vi "DriveControlManager.vi"(0 "Left Drive Manual Control":dbl, 1 "Right Drive Manual Control":dbl, 2 "left drive unit conversion (ticks/in)":dbl, 3 "right drive unit coversion (ticks/in)":dbl, 4 "LeftTrajectory":T1[](array[typedef]), 5 "RightTrajectory":T1[](array[typedef]), 6 "StartAtZero":bool=TRUE, 8 "Right Drive Motor DevRef":T3={"DeviceStatus"={"status"=FALSE, "code"=0, "source"=""}, "Type"=enum."PWM", "PWM"={"PWM Channel"=enum."PWM 1", "DeadBand"={"Name"="", "maxPositivePwm"=0, "minPositivePwm"=0, "centerPwm"=0, "maxNegativePwm"=0, "minNegativePwm"=0, "angularRange"=0}}, "CAN"={"Device Number"=0, "SetOutput VI Ref"=variant(enum8{"Percent VBus", "Current", "Speed", "Position", "Voltage"} enum."Percent VBus"), "GetOutput VI Ref"=variant(refnum<k1> refnum), "Enable VI Ref"=variant(dbl 12.0), "Disable VI Ref"=variant(enum8{"Percent VBus", "Speed", "Position", "Slave", "Unchanged / Invalid", "Voltage Compensation", "Current", "Motion Profile"} enum."Percent VBus"), "Data"=variant}, "Invert"=FALSE, "DIO PWM"={"PWM \"Enable\" Channel"=enum."Invalid", "DIOChannel"=enum."Invalid", "PWM Rate"=0.0}}, 9 "New Motion Profile":bool, 10 "Left Drive Motor DevRef":T3={"DeviceStatus"={"status"=FALSE, "code"=0, "source"=""}, "Type"=enum."PWM", "PWM"={"PWM Channel"=enum."PWM 1", "DeadBand"={"Name"="", "maxPositivePwm"=0, "minPositivePwm"=0, "centerPwm"=0, "maxNegativePwm"=0, "minNegativePwm"=0, "angularRange"=0}}, "CAN"={"Device Number"=0, "SetOutput VI Ref"=variant(enum8{"Percent VBus", "Current", "Speed", "Position", "Voltage"} enum."Percent VBus"), "GetOutput VI Ref"=variant(refnum<k1> refnum), "Enable VI Ref"=variant(dbl 12.0), "Disable VI Ref"=variant(enum8{"Percent VBus", "Speed", "Position", "Slave", "Unchanged / Invalid", "Voltage Compensation", "Current", "Motion Profile"} enum."Percent VBus"), "Data"=variant}, "Invert"=FALSE, "DIO PWM"={"PWM \"Enable\" Channel"=enum."Invalid", "DIOChannel"=enum."Invalid", "PWM Rate"=0.0}}) -> (14 "Drive Control State":T2)   [LabVIEW 2017]
uses:
  General/MotionProfiling/TypeDefs/MotionProfileControlState.ctl
  <vilib>/Rock Robotics/WPI/MotorControl/WPI_MotorControlDeviceRef.ctl
  <vilib>/Rock Robotics/WPI/MotorControl/WPI_MotorControlType.ctl
  <vilib>/Rock Robotics/SystemInterfaces/DIO/FPGA_DIOPWMChannel.ctl
  <vilib>/Rock Robotics/WPI/PWM/WPI_PWMDeadband.ctl
  <vilib>/Rock Robotics/SystemInterfaces/DIO/FPGA_DIOChannel.ctl
  Pathfinder/Pathfinder-LabVIEW/Pathfinder-Lib/VIs/Segment.ctl
  <vilib>/Rock Robotics/WPI/DriverStation/WPI_DriverStationRobotMode2.ctl
  ArgosLib/Signal Processing/TypeDefs/EdgeDetector_Type.ctl
  <vilib>/Rock Robotics/WPI/ThirdParty/Phoenix-LabVIEW/Motor Controller/Controls/CTRE_Phoenix_MotorControl_ControlMode.ctl
  Global_Var-RefNum/MotionProfileControlData.vi
  <vilib>/Rock Robotics/WPI/ThirdParty/Phoenix-LabVIEW/Motor Controller/Get/CTRE_Phoenix_MotorController_GetSelectedSensorData.vi
  <vilib>/Rock Robotics/WPI/ThirdParty/Phoenix-LabVIEW/Motor Controller/Get/CTRE_Phoenix_MotorController_GetClosedLoopData.vi
  <vilib>/Rock Robotics/WPI/ThirdParty/Phoenix-LabVIEW/Motor Controller/Get/CTRE_Phoenix_MotorController_GetVoltage.vi
  ArgosLib/ArgosLib.lvlib
  Pathfinder/Pathfinder-LabVIEW/Pathfinder-Lib/Pathfinder.lvlib
panel:
  in  "StopDetectTime (ms)":u32
  in  "Tab Control":enum32{"I/O", "Calibration", "Status"}(tab)
  in  "ClearMotionProfile":bool
  out "Max Left Drive Speed (Sensor Units per 100 ms)":i32
  out "Max Right Drive Speed (Sensor Units per 100 ms)":i32
  in  "Reset Right Drive Max":bool
  in  "Reset Left Drive Max":bool
  in  "Reset Left Drive Sensor":bool
  in  "Reset Right Drive Sensor":bool
  in  "Left Drive Position (in)":dbl
  in  "Right Drive Position (in)":dbl
  out "Left Drive":T8
  out "Right Drive":T8
  out "RightDriveFaults":T9
  out "LeftDriveFaults":T9
  out "Right Error":i32
  out "Left Error":i32
  out "LeftDriveV":dbl(graph)
  out "RightDriveV":dbl(graph)
  out "Right Drive":T8(graph)
  out "Left Drive":T8(graph)
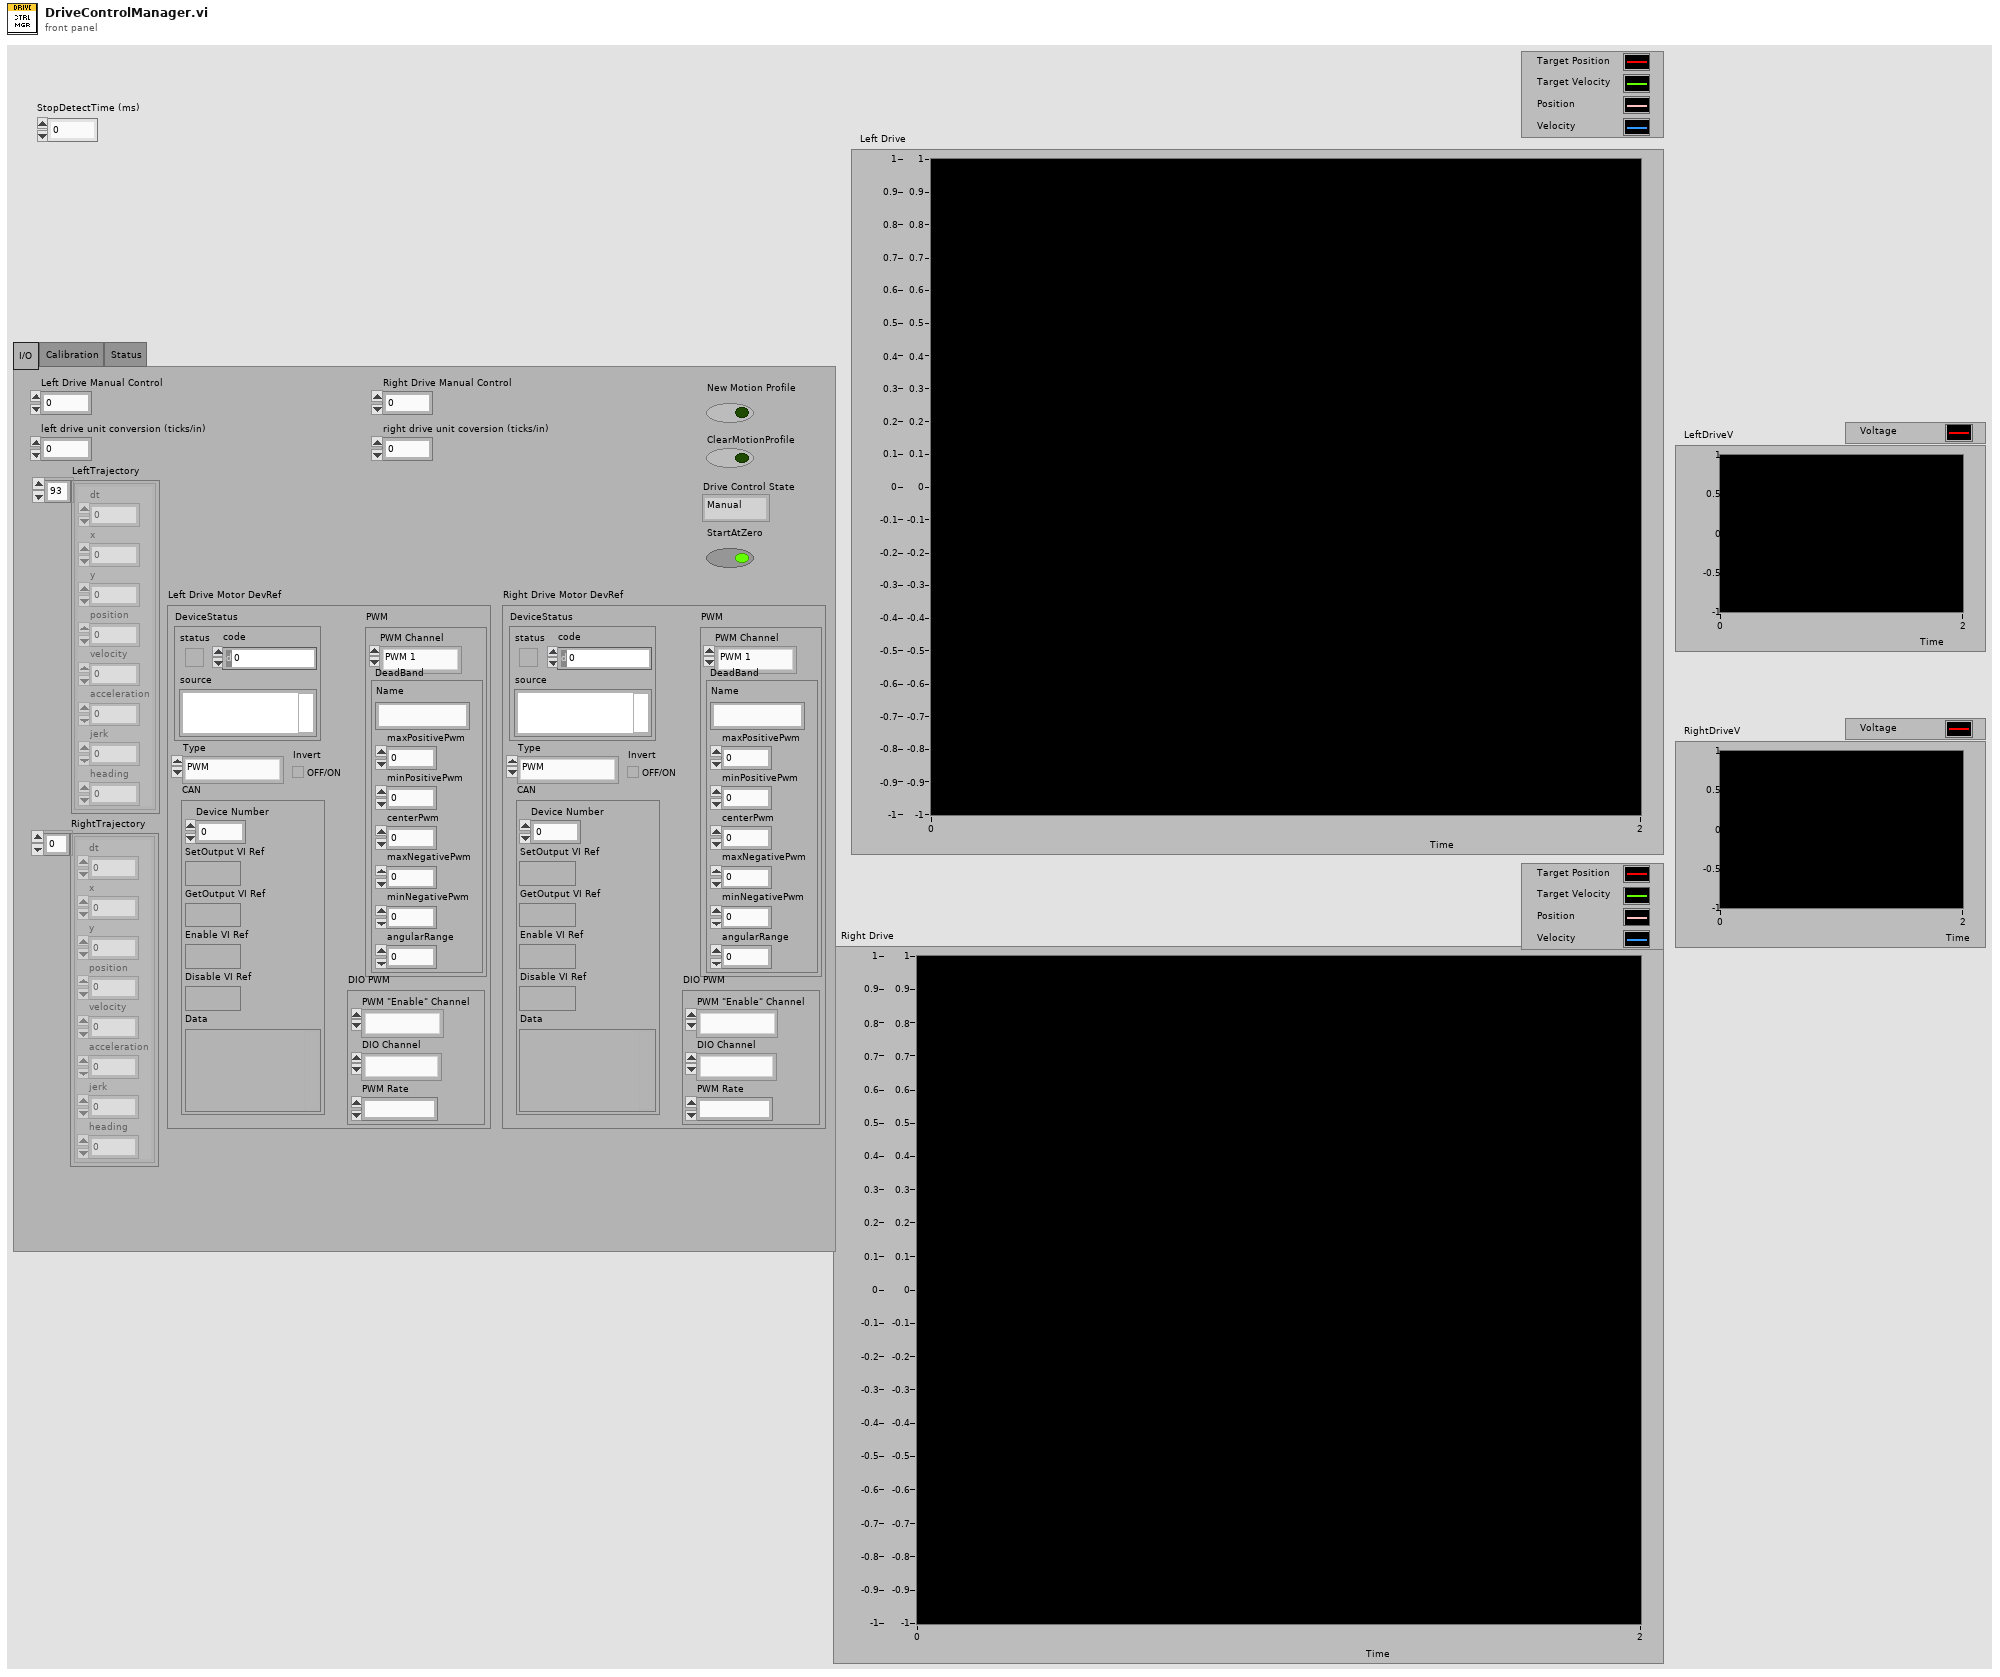
[diagram p1: front panel]
types:
  T1 = typedef "Pathfinder.lvlib/Segment.ctl" = cluster{"dt":dbl, "x":dbl, "y":dbl, "position":dbl, "velocity":dbl, "acceleration":dbl, "jerk":dbl, "heading":dbl}
  T2 = typedef "MotionProfileControlState.ctl" = enum16{"Manual", "Auto_Idle", "Auto_Run"}
  T3 = typedef "WPI_MotorControlDeviceRef.ctl" = cluster{"DeviceStatus":errorcluster, "Type":T4, "PWM":cluster{"PWM Channel":T5, "DeadBand":T6}, "CAN":cluster{"Device Number":u8, "SetOutput VI Ref":variant, "GetOutput VI Ref":variant, "Enable VI Ref":variant, "Disable VI Ref":variant, "Data":variant}, "Invert":bool, "DIO PWM":cluster{"PWM \"Enable\" Channel":T5, "DIOChannel":T7, "PWM Rate":dbl}}
  T4 = typedef "WPI_MotorControlType.ctl" = enum16{"PWM", "CAN", "DIO PWM"}
  T5 = typedef "FPGA_DIOPWMChannel.ctl" = enum8{"PWM 0", "PWM 1", "PWM 2", "PWM 3", "PWM 4", "PWM 5", "PWM 6", "PWM 7", "PWM 8", "PWM 9", "PWM MXP 0", "PWM MXP 1", "PWM MXP 2", "PWM MXP 3", "PWM MXP 4", "PWM MXP 5", "PWM MXP 6", "PWM MXP 7", "PWM MXP 8", "PWM MXP 9", "Invalid"}
  T6 = typedef "WPI_PWMDeadband.ctl" = cluster{"Name":string, "maxPositivePwm":i32, "minPositivePwm":i32, "centerPwm":i32, "maxNegativePwm":i32, "minNegativePwm":i32, "angularRange":u16}
  T7 = typedef "FPGA_DIOChannel.ctl" = enum8{"DIO 0", "DIO 1", "DIO 2", "DIO 3", "DIO 4", "DIO 5", "DIO 6", "DIO 7", "DIO 8", "DIO 9", "DIO MXP 0", "DIO MXP 1", "DIO MXP 2", "DIO MXP 3", "DIO MXP 4", "DIO MXP 5", "DIO MXP 6", "DIO MXP 7", "DIO MXP 8", "DIO MXP 9", "DIO MXP 10", "DIO MXP 11", "DIO MXP 12", "DIO MXP 13", "DIO MXP 14", "DIO MXP 15", "SPI Port CS1", "SPI Port CS2", "SPI Port CS3", "SPI Port MISO", "SPI Port MOSI", "Invalid"}
  T8 = cluster{"Position (Sensor Units)":i32, "Velocity (Sensor Units per 100 ms)":i32, "Position (Raw Sensor Units)":i32, "Velocity (Raw Sensor Units per 100 ms)":i32}
  T9 = cluster{"Under Voltage":bool, "Forward Limit Switch":bool, "Reverse Limit Switch":bool, "Forward Soft Limit":bool, "Reverse Soft Limit":bool, "Hardware Failure":bool, "Reset During Enable":bool, "Sensor Overflow":bool, "Sensor Out of Phase":bool, "Hardware ESD Reset":bool, "Remote Loss of Signal":bool}
  T10 = typedef "WPI_DriverStationRobotMode2.ctl" = enum16{"Autonomous Disabled", "Autonomous Enabled", "Teleop Disabled", "Teleop Enabled", "Disconnected", "Finish", "Test Disabled", "Test Enabled", "Emergency Stopped"}
  T11 = typedef "ArgosLib.lvlib/EdgeDetector_Type.ctl" = enum16{"RisingEdge", "FallingEdge", "Both"}
  T12 = cluster{"Position (Sensor Units)":i32, "Velocity (Sensor Units per 100 ms)":i32, "Position (Raw Sensor Units)":i32, "Velocity (Raw Sensor Units per 100 ms)":i32}[]
  T13 = typedef "CTRE_Phoenix_MotorControl_ControlMode.ctl" = u16
  T14 = typedef "DriveMotionProfileControl.ctl" = cluster{"ControlMutex":T15, "Trajectory Points":T1[], "CurrentIndex":u32}
  T15 = typedef "Semaphore RefNum" = refnum<k1>
  T16 = cluster{"Position (Raw Sensor Units)":i32, "Closed-loop Target":i32, "Position (Raw Sensor Units)":i32, "Velocity (Raw Sensor Units per 100 ms)":i32}
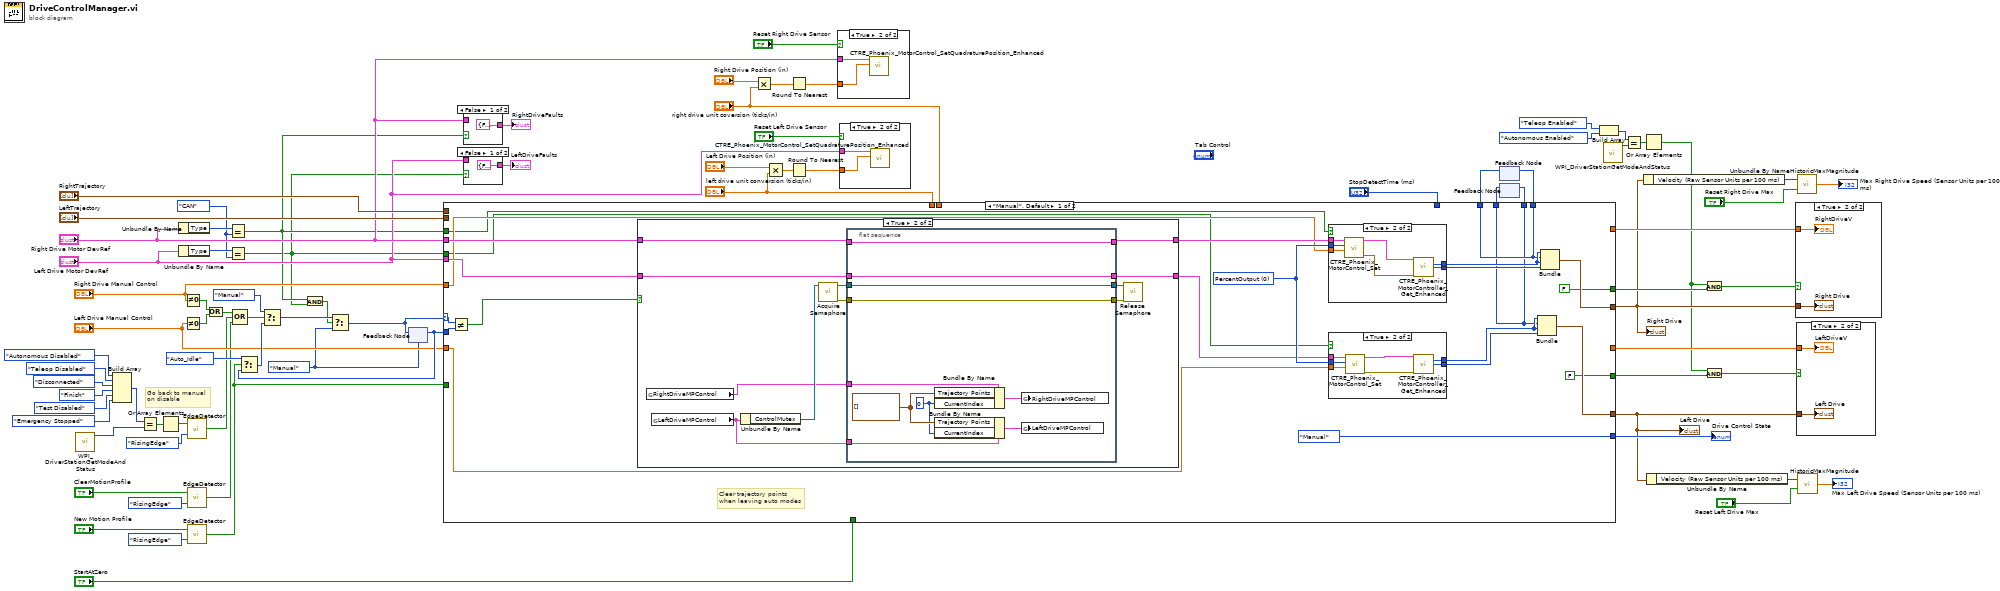
[diagram p0: block diagram]
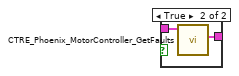
[diagram p2: hidden frame]
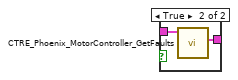
[diagram p3: hidden frame]
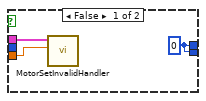
[diagram p8: hidden frame]
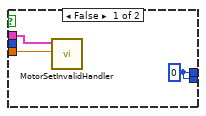
[diagram p9: hidden frame]
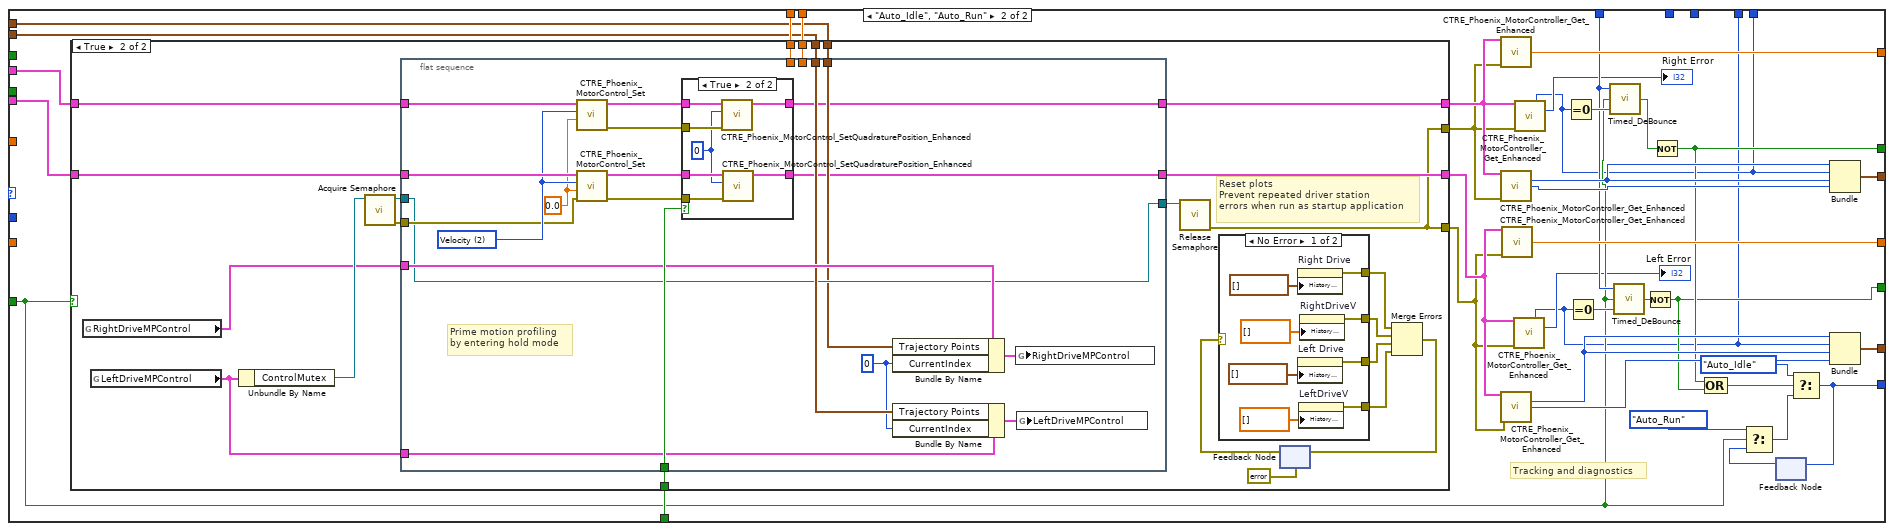
[diagram p11: hidden frame]
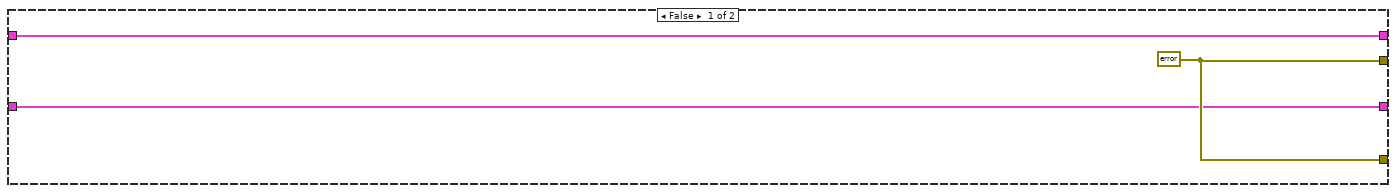
[diagram p12: hidden frame]
diagram:
  w4 = MotionProfileControlState."Manual" ("f")
  w7 = WPI_MotorControlType."CAN" ("y")
  # "Go back to manual\non disable"
  n1 = call <vilib>:"WPI_DriverStationGetModeAndStatus.vi"() -> ("Robot Mode"=w39:T10)  [unwired: 10 in, 1 out]
  n2 = Build Array(WPI_DriverStationRobotMode2."Autonomous Disabled" ("Robot Mode"), WPI_DriverStationRobotMode2."Teleop Disabled" ("Robot Mode"), WPI_DriverStationRobotMode2."Disconnected" ("Robot Mode"), WPI_DriverStationRobotMode2."Finish" ("Robot Mode"), WPI_DriverStationRobotMode2."Test Disabled" ("Robot Mode"), WPI_DriverStationRobotMode2."Emergency Stopped" ("Robot Mode")) -> (w40:T10[])
  n3 = Equal?(x=w40, y=w39) -> (x = y?=w38:bool[])
  n4 = Or Array Elements(Boolean array=w38) -> (logical OR=w37:bool)
  n5 = Unbundle By Name("Right Drive Motor DevRef") -> ("Type"=w9:T4)
  n6 = Unbundle By Name("Left Drive Motor DevRef") -> ("Type"=w8:T4)
  n7 = Not Equal To 0?(x="Right Drive Manual Control") -> (x != 0?=w80:bool)
  n8 = Not Equal To 0?(x="Left Drive Manual Control") -> (x != 0?=w79:bool)
  n9 = call "EdgeDetector.vi"("DetectorType"=EdgeDetector_Type."RisingEdge", "Input"=w37) -> ("Edge"=w34:bool)
  n10 = call "EdgeDetector.vi"("DetectorType"=EdgeDetector_Type."RisingEdge", "Input"="ClearMotionProfile") -> ("Edge"=w35:bool)
  n11 = call "EdgeDetector.vi"("DetectorType"=EdgeDetector_Type."RisingEdge", "Input"="New Motion Profile") -> ("Edge"=w72:bool)
  n12 = Or(x=w80, y=w79) -> (x .or. y?=w55:bool)
  n13 = Equal?(x=w9, y=w7) -> (x = y?=w2:bool)
  n14 = Equal?(x=w8, y=w7) -> (x = y?=w1:bool)
  n15 = Compound Arithmetic op=OR(w55, w34, w35) -> (w56:bool)
  n16 = And(x=w2, y=w1) -> (x .and. y?=w3:bool)
  n17 = feedback #1(w4) -> (w76:T2)
  n18 = Select(t=MotionProfileControlState."Auto_Idle", s=w72, f=w76) -> (s? t:f=w77:T2)
  n19 = Select(t=MotionProfileControlState."Manual" ("Arm Control State"), s=w56, f=w77) -> (s? t:f=w6:T2)
  n20 = Select(t=w6, s=w3, f=w4) -> (s? t:f=w5:T2)
  n21 = feedback-in #1(w5) -> ()
  n22 = case shown="False" w2 {
    tunnel: [T9 {"Under Voltage"=FALSE, "Forward Limit Switch"=FALSE, "Reverse Limit Switch"=FALSE, "Forward Soft Limit"=FALSE, "Reverse Soft Limit"=FALSE, "Hardware Failure"=FALSE, "Reset During Enable"=FALSE, "Sensor Overflow"=FALSE, "Sensor Out of Phase"=FALSE, "Hardware ESD Reset"=FALSE, "Remote Loss of Signal"=FALSE} ("Faults") w83] -> w70
    tunnel: "Right Drive Motor DevRef" -> [_ w82]
    frame False {
    }
    frame True {
      n23 = call <vilib>:"CTRE_Phoenix_MotorController_GetFaults.vi"("PhoenixMotorControlDevRef"=w82) -> ("Faults"=w83:T9)  [unwired: 8 in, 2 out]
    }
  }
  "RightDriveFaults" <- w70
  n24 = case shown="False" w1 {
    tunnel: [T9 {"Under Voltage"=FALSE, "Forward Limit Switch"=FALSE, "Reverse Limit Switch"=FALSE, "Forward Soft Limit"=FALSE, "Reverse Soft Limit"=FALSE, "Hardware Failure"=FALSE, "Reset During Enable"=FALSE, "Sensor Overflow"=FALSE, "Sensor Out of Phase"=FALSE, "Hardware ESD Reset"=FALSE, "Remote Loss of Signal"=FALSE} ("Faults") w86] -> w67
    tunnel: "Left Drive Motor DevRef" -> [_ w85]
    frame False {
    }
    frame True {
      n25 = call <vilib>:"CTRE_Phoenix_MotorController_GetFaults.vi"("PhoenixMotorControlDevRef"=w85) -> ("Faults"=w86:T9)  [unwired: 8 in, 2 out]
    }
  }
  "LeftDriveFaults" <- w67
  n26 = Multiply(x="Right Drive Position (in)", y="right drive unit coversion (ticks/in)") -> (x*y=w50:dbl)
  n27 = Multiply(x="Left Drive Position (in)", y="left drive unit conversion (ticks/in)") -> (x*y=w53:dbl)
  n28 = Round To Nearest(number=w50) -> (nearest integer value=w49:dbl)
  n29 = Round To Nearest(number=w53) -> (nearest integer value=w52:dbl)
  n30 = case shown="True" "Reset Right Drive Sensor" {
    tunnel: "Right Drive Motor DevRef" -> [_ w88]
    tunnel: w49 -> [_ w87]
    frame False {
    }
    frame True {
      n31 = call <vilib>:"CTRE_Phoenix_MotorControl_SetQuadraturePosition_Enhanced.vi"("New Position"=w87, "PhoenixMotorControlDevRef"=w88) -> ()  [unwired: 8 in, 2 out]
    }
  }
  n32 = case shown="True" "Reset Left Drive Sensor" {
    tunnel: "Left Drive Motor DevRef" -> [_ w90]
    tunnel: w52 -> [_ w89]
    frame False {
    }
    frame True {
      n33 = call <vilib>:"CTRE_Phoenix_MotorControl_SetQuadraturePosition_Enhanced.vi"("New Position"=w89, "PhoenixMotorControlDevRef"=w90) -> ()  [unwired: 8 in, 2 out]
    }
  }
  n34 = feedback #2() -> (w15:i32)  [unwired: 1 in]
  n35 = feedback #3() -> (w14:i32)  [unwired: 1 in]
  n36 = case shown="\"Manual\", Default" w5 {
    selector: w5 -> [w111 _]
    tunnel: "Right Drive Motor DevRef" -> [w108 w193]
    tunnel: "Left Drive Motor DevRef" -> [w106 w192]
    tunnel: "Right Drive Manual Control" -> [w97 _]
    tunnel: "Left Drive Manual Control" -> [w112 _]
    tunnel: w76 -> [w110 _]
    tunnel: w72 -> [_ w164]
    tunnel: "RightTrajectory" -> [_ w177]
    tunnel: "LeftTrajectory" -> [_ w178]
    tunnel: [MotionProfileControlState."Manual" ("Arm Control State") w185] -> w71
    tunnel: [w103 w189] -> w48
    tunnel: [w100 w188] -> w47
    tunnel: [FALSE w162] -> w61
    tunnel: [FALSE w161] -> w64
    tunnel: [_ w187] -> w58
    tunnel: [_ w186] -> w57
    tunnel: "left drive unit conversion (ticks/in)" -> [_ w179]
    tunnel: "right drive unit coversion (ticks/in)" -> [_ w180]
    tunnel: "StartAtZero" -> [_ w181]
    tunnel: "StopDetectTime (ms)" -> [_ w165]
    tunnel: [w94 w158] -> w17
    tunnel: [w93 w157] -> w16
    tunnel: w15 -> [w94 _]
    tunnel: w14 -> [w93 _]
    tunnel: w2 -> [w92 _]
    tunnel: w1 -> [w91 _]
    frame "Manual", Default {
      w113 = T13 0 items=["PercentOutput"=0, "Position"=1, "Velocity"=2, "Current"=3, "Follower"=5, "MotionProfile"=6, "MotionMagic"=7, "MotionMagicArc"=8, "MotionProfileArc"=10, "Disabled"=15] ("Control Mode")
      # "Clear trajectory points\nwhen leaving auto modes"
      n37 = Not Equal?(x=w111, y=w110) -> (x != y?=w109:bool)
      n38 = case shown="True" w109 {
        tunnel: w108 -> [w135 w146]
        tunnel: [w135 w145] -> w107
        tunnel: w106 -> [w134 w144]
        tunnel: [w134 w143] -> w105
        frame False {
        }
        frame True {
          n39 = global read "MotionProfileControlData.vi" "RightDriveMPControl"() -> (w139:T14)
          n40 = global read "MotionProfileControlData.vi" "LeftDriveMPControl"() -> (w138:T14)
          n41 = Unbundle By Name(w138) -> ("ControlMutex"=w141:T15)
          n42 = call <vilib>:"Acquire Semaphore.vi"("semaphore"=w141) -> ("error out"=w142:errorcluster, "semaphore out"=w137:T15)  [unwired: 4 in, 1 out]
          n43 = flat-sequence {
            tunnel: w146 -> [w156]
            tunnel: [w156] -> w145
            tunnel: w144 -> [w155]
            tunnel: [w155] -> w143
            tunnel: w142 -> [w154]
            tunnel: [w154] -> w140
            tunnel: w139 -> [w153]
            tunnel: w138 -> [w152]
            tunnel: [w147] -> w136
            tunnel: w137 -> [w147]
            frame #0 {
              w150 = u32 0 ("CurrentIndex")
              w151 = T1[] [] ("Trajectory Points")
              n44 = Bundle By Name(cluster=w153, "Trajectory Points"=w151, "CurrentIndex"=w150) -> (w148:T14)
              n45 = Bundle By Name(cluster=w152, "Trajectory Points"=w151, "CurrentIndex"=w150) -> (w149:T14)
              n46 = global write "MotionProfileControlData.vi" "RightDriveMPControl"(w148) -> ()
              n47 = global write "MotionProfileControlData.vi" "LeftDriveMPControl"(w149) -> ()
            }
          }
          n48 = call <vilib>:"Release Semaphore.vi"("error in (no error)"=w140, "semaphore"=w136) -> ()  [unwired: 4 in, 2 out]
        }
      }
      n49 = case shown="True" w92 {
        tunnel: w113 -> [_ w133]
        tunnel: w107 -> [w126 w132]
        tunnel: [w124 w131] -> w102
        tunnel: w97 -> [w125 w130]
        tunnel: [w124 w127] -> w95
        frame False {
          w124 = 0 ("Position (Raw Sensor Units)")
          n50 = call "MotorSetInvalidHandler.vi"("Output"=w125, "MotorControlDevRef"=w126) -> ()  [unwired: 7 in, 3 out]
        }
        frame True {
          n51 = call <vilib>:"CTRE_Phoenix_MotorControl_Set.vi"("Output"=w130, "Control Mode"=w133, "PhoenixMotorControlDevRef"=w132) -> ("error out"=w128:errorcluster, "PhoenixMotorControlDevRef"=w129:T3)  [unwired: 7 in]
          n52 = call-poly <vilib>:"CTRE_Phoenix_MotorController_Get_Enhanced.vi"("PhoenixMotorControlDevRef"=w129, "error in"=w128) -> ("Position (Raw Sensor Units)"=w127:i32, "Velocity (Raw Sensor Units per 100 ms)"=w131:i32)  [unwired: 10 in, 2 out]
        }
      }
      n53 = case shown="True" w91 {
        tunnel: w113 -> [_ w123]
        tunnel: w112 -> [w115 w122]
        tunnel: w105 -> [w116 w121]
        tunnel: [w114 w120] -> w101
        tunnel: [w114 w117] -> w96
        frame False {
          w114 = 0 ("Position (Raw Sensor Units)")
          n54 = call "MotorSetInvalidHandler.vi"("Output"=w115, "MotorControlDevRef"=w116) -> ()  [unwired: 7 in, 3 out]
        }
        frame True {
          n55 = call <vilib>:"CTRE_Phoenix_MotorControl_Set.vi"("Output"=w122, "Control Mode"=w123, "PhoenixMotorControlDevRef"=w121) -> ("error out"=w118:errorcluster, "PhoenixMotorControlDevRef"=w119:T3)  [unwired: 7 in]
          n56 = call-poly <vilib>:"CTRE_Phoenix_MotorController_Get_Enhanced.vi"("PhoenixMotorControlDevRef"=w119, "error in"=w118) -> ("Position (Raw Sensor Units)"=w117:i32, "Velocity (Raw Sensor Units per 100 ms)"=w120:i32)  [unwired: 10 in, 2 out]
        }
      }
      n57 = Bundle("Position (Raw Sensor Units)"=w96, "Closed-loop Target"=w93, "Position (Raw Sensor Units)"=w96, "Velocity (Raw Sensor Units per 100 ms)"=w101) -> (w100:T16)  [unwired: 1 in]
      n58 = Bundle("Position (Raw Sensor Units)"=w95, "Closed-loop Target"=w94, "Position (Raw Sensor Units)"=w95, "Velocity (Raw Sensor Units per 100 ms)"=w102) -> (w103:T16)  [unwired: 1 in]
    }
    frame "Auto_Idle", "Auto_Run" {
      # "Tracking and diagnostics"
      n59 = case shown="True" w164 {
        tunnel: w193 -> [w195 w219]
        tunnel: w192 -> [w194 w218]
        tunnel: [w195 w206] -> w169
        tunnel: [w194 w205] -> w173
        tunnel: w181 -> [_ w217]
        tunnel: w180 -> [_ w214]
        tunnel: w179 -> [_ w213]
        tunnel: w177 -> [_ w210]
        tunnel: w178 -> [_ w209]
        tunnel: [w196 w204] -> w168
        tunnel: [w196 w204] -> w172
        frame False {
          w196 = errorcluster {"status"=FALSE, "code"=0, "source"=""} ("error out")
        }
        frame True {
          # "Reset plots\nPrevent repeated driver station\nerrors when run as startup application"
          n60 = global read "MotionProfileControlData.vi" "RightDriveMPControl"() -> (w212:T14)
          n61 = global read "MotionProfileControlData.vi" "LeftDriveMPControl"() -> (w211:T14)
          n62 = Unbundle By Name(w211) -> ("ControlMutex"=w215:T15)
          n63 = call <vilib>:"Acquire Semaphore.vi"("semaphore"=w215) -> ("error out"=w216:errorcluster, "semaphore out"=w208:T15)  [unwired: 4 in, 1 out]
          n64 = flat-sequence {
            tunnel: w219 -> [w248]
            tunnel: w218 -> [w247]
            tunnel: w217 -> [w244]
            tunnel: w216 -> [w243]
            tunnel: w214 -> [_]
            tunnel: w213 -> [_]
            tunnel: [w234] -> w206
            tunnel: [w235] -> w205
            tunnel: w212 -> [w242]
            tunnel: w211 -> [w241]
            tunnel: w210 -> [w236]
            tunnel: w209 -> [w240]
            tunnel: w208 -> [w237]
            tunnel: [w237] -> w207
            frame #0 {
              w233 = u32 0 ("CurrentIndex")
              w245 = 0.0 ("Output")
              w246 = T13 2 items=["PercentOutput"=0, "Position"=1, "Velocity"=2, "Current"=3, "Follower"=5, "MotionProfile"=6, "MotionMagic"=7, "MotionMagicArc"=8, "MotionProfileArc"=10, "Disabled"=15] ("Control Mode")
              # "Prime motion profiling\nby entering hold mode"
              n65 = call <vilib>:"CTRE_Phoenix_MotorControl_Set.vi"("Output"=w245, "Control Mode"=w246, "PhoenixMotorControlDevRef"=w248) -> ("error out"=w231:errorcluster, "PhoenixMotorControlDevRef"=w232:T3)  [unwired: 7 in]
              n66 = call <vilib>:"CTRE_Phoenix_MotorControl_Set.vi"("error in (no error)"=w243, "Output"=w245, "Control Mode"=w246, "PhoenixMotorControlDevRef"=w247) -> ("error out"=w229:errorcluster, "PhoenixMotorControlDevRef"=w230:T3)  [unwired: 6 in]
              n67 = case shown="True" w244 {
                tunnel: w232 -> [w250 w257]
                tunnel: w230 -> [w249 w255]
                tunnel: w229 -> [_ w254]
                tunnel: w231 -> [_ w256]
                tunnel: [w250 w253] -> w234
                tunnel: [w249 w252] -> w235
                frame False {
                }
                frame True {
                  w251 = 0 ("New Position")
                  n68 = call <vilib>:"CTRE_Phoenix_MotorControl_SetQuadraturePosition_Enhanced.vi"("error in (no error)"=w256, "New Position"=w251, "PhoenixMotorControlDevRef"=w257) -> ("PhoenixMotorControlDevRef"=w253:T3)  [unwired: 7 in, 1 out]
                  n69 = call <vilib>:"CTRE_Phoenix_MotorControl_SetQuadraturePosition_Enhanced.vi"("error in (no error)"=w254, "New Position"=w251, "PhoenixMotorControlDevRef"=w255) -> ("PhoenixMotorControlDevRef"=w252:T3)  [unwired: 7 in, 1 out]
                }
              }
              n70 = Bundle By Name(cluster=w242, "Trajectory Points"=w236, "CurrentIndex"=w233) -> (w239:T14)
              n71 = Bundle By Name(cluster=w241, "Trajectory Points"=w240, "CurrentIndex"=w233) -> (w238:T14)
              n72 = global write "MotionProfileControlData.vi" "RightDriveMPControl"(w239) -> ()
              n73 = global write "MotionProfileControlData.vi" "LeftDriveMPControl"(w238) -> ()
            }
          }
          n74 = call <vilib>:"Release Semaphore.vi"("semaphore"=w207) -> ("error out"=w204:errorcluster)  [unwired: 5 in, 1 out]
          n75 = feedback #4(errorcluster {"status"=FALSE, "code"=0, "source"=""} ("error IO")) -> (w198:errorcluster)
          n76 = case shown="No Error" w198 {
            selector: w198 -> [_ w228]
            tunnel: [w223 w228] -> w203
            tunnel: [w222 w228] -> w202
            tunnel: [w221 w228] -> w201
            tunnel: [w220 w228] -> w200
            frame No Error {
              n77 = property on="Right Drive" class="WFChart (strict)"("History Data"=T12 []) -> (error out=w223:errorcluster)  [unwired: 2 in, 1 out]
              n78 = property on="Left Drive" class="WFChart (strict)"("History Data"=T12 []) -> (error out=w221:errorcluster)  [unwired: 2 in, 1 out]
              n79 = property on="LeftDriveV" class="WFChart (strict)"("History Data"=dbl[] []) -> (error out=w220:errorcluster)  [unwired: 2 in, 1 out]
              n80 = property on="RightDriveV" class="WFChart (strict)"("History Data"=dbl[] []) -> (error out=w222:errorcluster)  [unwired: 2 in, 1 out]
            }
            frame Error {
            }
          }
          n81 = Merge Errors(w203, w202, w201, w200) -> (w199:errorcluster)
          n82 = feedback-in #4(w199) -> ()
        }
      }
      n83 = call-poly <vilib>:"CTRE_Phoenix_MotorController_Get_Enhanced.vi"("PhoenixMotorControlDevRef"=w169, "error in"=w168) -> ("Output Voltage"=w186:dbl)  [unwired: 9 in, 4 out]
      n84 = call-poly <vilib>:"CTRE_Phoenix_MotorController_Get_Enhanced.vi"("PhoenixMotorControlDevRef"=w169, "error in"=w168) -> ("Position (Raw Sensor Units)"=w167:i32, "Velocity (Raw Sensor Units per 100 ms)"=w175:i32)  [unwired: 10 in, 2 out]
      n85 = call-poly <vilib>:"CTRE_Phoenix_MotorController_Get_Enhanced.vi"("PhoenixMotorControlDevRef"=w173, "error in"=w172) -> ("Position (Raw Sensor Units)"=w174:i32, "Velocity (Raw Sensor Units per 100 ms)"=w176:i32)  [unwired: 10 in, 2 out]
      n86 = call-poly <vilib>:"CTRE_Phoenix_MotorController_Get_Enhanced.vi"("PhoenixMotorControlDevRef"=w173, "error in"=w172) -> ("Output Voltage"=w187:dbl)  [unwired: 9 in, 4 out]
      n87 = call-poly <vilib>:"CTRE_Phoenix_MotorController_Get_Enhanced.vi"("PhoenixMotorControlDevRef"=w173, "error in"=w172) -> ("Closed-loop Target"=w157:i32, "Closed-loop Error"=→"Left Error":i32)  [unwired: 8 in, 4 out]
      n88 = call-poly <vilib>:"CTRE_Phoenix_MotorController_Get_Enhanced.vi"("PhoenixMotorControlDevRef"=w169, "error in"=w168) -> ("Closed-loop Target"=w158:i32, "Closed-loop Error"=→"Right Error":i32)  [unwired: 8 in, 4 out]
      n89 = Equal To 0?(x=w158) -> (x = 0?=w166:bool)
      n90 = Equal To 0?(x=w157) -> (x = 0?=w171:bool)
      n91 = call "Timed_DeBounce.vi"("Input"=w166, "Reset"=w164, "Hold Time(ms)"=w165) -> ("Output"=w163:bool)
      n92 = call "Timed_DeBounce.vi"("Input"=w171, "Reset"=w164, "Hold Time(ms)"=w165) -> ("Output"=w170:bool)
      n93 = Not(x=w170) -> (.not. x?=w161:bool)
      n94 = Not(x=w163) -> (.not. x?=w162:bool)
      n95 = Compound Arithmetic op=OR(w162, w161) -> (w191:bool)
      n96 = feedback #5() -> (w182:T2)  [unwired: 1 in]
      n97 = Select(t=MotionProfileControlState."Auto_Run" ("Arm Control State"), s=w164, f=w182) -> (s? t:f=w183:T2)
      n98 = Select(t=MotionProfileControlState."Auto_Idle" ("Arm Control State"), s=w191, f=w183) -> (s? t:f=w185:T2)
      n99 = feedback-in #5(w185) -> ()
      n100 = Bundle("Position (Raw Sensor Units)"=w167, "Closed-loop Target"=w158, "Position (Raw Sensor Units)"=w167, "Velocity (Raw Sensor Units per 100 ms)"=w175) -> (w189:T16)  [unwired: 1 in]
      n101 = Bundle("Position (Raw Sensor Units)"=w174, "Closed-loop Target"=w157, "Position (Raw Sensor Units)"=w174, "Velocity (Raw Sensor Units per 100 ms)"=w176) -> (w188:T16)  [unwired: 1 in]
    }
  }
  "Drive Control State" <- w71
  "Right Drive" <- w48
  "Left Drive" <- w47
  n102 = feedback-in #2(w17) -> ()
  n103 = feedback-in #3(w16) -> ()
  n104 = Build Array(WPI_DriverStationRobotMode2."Teleop Enabled" ("Robot Mode"), WPI_DriverStationRobotMode2."Autonomous Enabled" ("Robot Mode")) -> (w27:T10[])
  n105 = call <vilib>:"WPI_DriverStationGetModeAndStatus.vi"() -> ("Robot Mode"=w60:T10)  [unwired: 10 in, 1 out]
  n106 = Equal?(x=w27, y=w60) -> (x = y?=w59:bool[])
  n107 = Unbundle By Name(w48) -> ("Velocity (Raw Sensor Units per 100 ms)"=w33:i32)
  n108 = Or Array Elements(Boolean array=w59) -> (logical OR=w26:bool)
  n109 = Unbundle By Name(w47) -> ("Velocity (Raw Sensor Units per 100 ms)"=w32:i32)
  n110 = And(x=w26, y=w61) -> (x .and. y?=w31:bool)
  n111 = And(x=w26, y=w64) -> (x .and. y?=w30:bool)
  n112 = case shown="True" w31 {
    tunnel: w48 -> [_ w259]
    tunnel: w57 -> [_ w258]
    frame False {
    }
    frame True {
      "Right Drive" <- w259
      "RightDriveV" <- w258
    }
  }
  n113 = case shown="True" w30 {
    tunnel: w47 -> [_ w261]
    tunnel: w58 -> [_ w260]
    frame False {
    }
    frame True {
      "Left Drive" <- w261
      "LeftDriveV" <- w260
    }
  }
  n114 = call "HistoricMaxMagnitude.vi"("Reset"="Reset Right Drive Max", "Value"=w33) -> ("Max"=→"Max Right Drive Speed (Sensor Units per 100 ms)":dbl)
  n115 = call "HistoricMaxMagnitude.vi"("Reset"="Reset Left Drive Max", "Value"=w32) -> ("Max"=→"Max Left Drive Speed (Sensor Units per 100 ms)":dbl)
